vi "Check Abort.vi"(8 "error in (no error)":errorcluster, 11 "Father of all uServices in":refnum<class "Father of all uServices.lvclass">) -> (0 "error out":errorcluster, 2 "Abort":bool, 3 "Father of all uServices out":refnum<class "Father of all uServices.lvclass">)   [LabVIEW 2020, in "TALOS.lvlib" / "Father of all uServices.lvlib" / "Father of all uServices.lvclass"]
uses:
  Father of all uServices.lvclass
  TALOS.lvlib
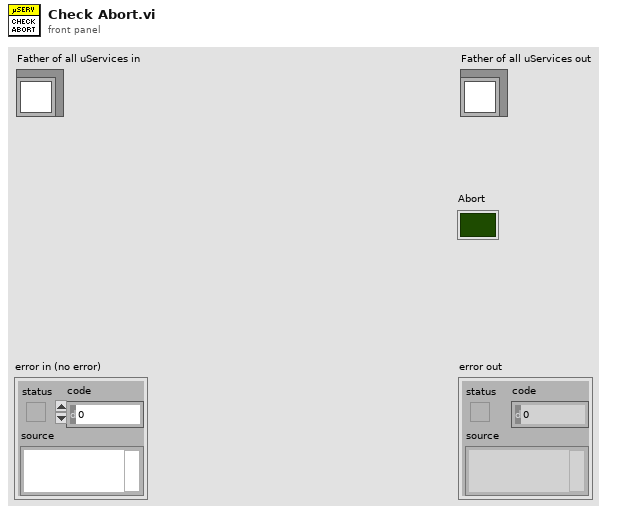
[diagram p1: front panel]
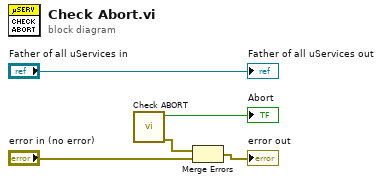
[diagram p0: block diagram]
diagram:
  n1 = call "Check ABORT.vi"() -> ("error out"=w1:errorcluster, "ABORT?"=→"Abort":bool)  [unwired: 10 in]
  n2 = Merge Errors(w1, "error in (no error)") -> (→"error out":errorcluster)
  "Father of all uServices out" <- "Father of all uServices in"
